vi "Get ADC Value from Entry.vi"(11 "Entries":T1[](array[typedef])) -> (3 "ADC Values":cluster{i32[]}[](array[cluster]))   [LabVIEW 2019, in "Muon Data Post-Processing.lvlib"]
uses:
  Muon Data Post-Processing.lvlib
  File Entry.ctl
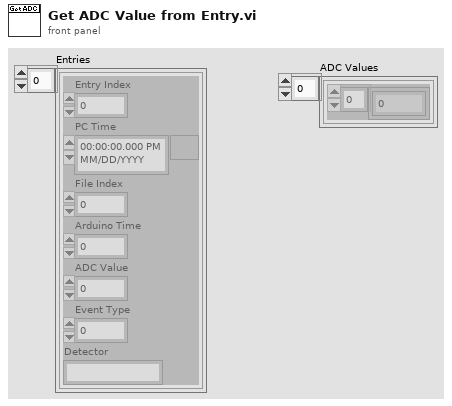
[diagram p1: front panel]
types:
  T1 = typedef "Muon Data Post-Processing.lvlib/File Entry.ctl" = cluster{"Entry Index":i32, "PC Time":timestamp, "File Index":i32, "Arduino Time":i32, "ADC Value":i32, "Event Type":i32, "Detector":string}
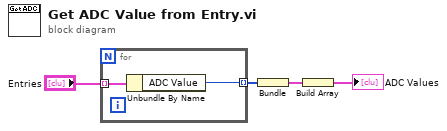
[diagram p0: block diagram]
diagram:
  n1 = for {
    tunnel: "Entries" -> [w6] mode=indexing
    tunnel: [w5] -> w3 mode=indexing
    n2 = Unbundle By Name(w6) -> ("ADC Value"=w5:i32)
  }
  n3 = Bundle(w3) -> (w2:cluster{i32[]})  [unwired: 1 in]
  n4 = Build Array(w2) -> (→"ADC Values":cluster{i32[]}[])
